vi "Get Modbus Channels.vi"(8 "error in (no error)":errorcluster, 10 "Chassis Name":tag, 11 "TimingGrp.lvclass":refnum<class "TimingGrp.lvclass">) -> (0 "error out":errorcluster, 1 "Num of Chans":i32, 3 "All Rate MB Chans":string[](array[string]))   [LabVIEW 2018, in "Configuration Grandmaster.lvlib" / "TimingGrp.lvclass"]
uses:
  TimingGrp.lvclass
  TimingGrp.lvclass/TimingGrp.ctl
  Class Chan Group/Read GroupChans.vi
  Measurements/Class Channel/Read ChanName.vi
  Measurements/Class Channel/Read ToModBus.vi
  Measurements/Class Channel/Channel.lvclass
  Class Chan Group/ChanGrp.lvclass
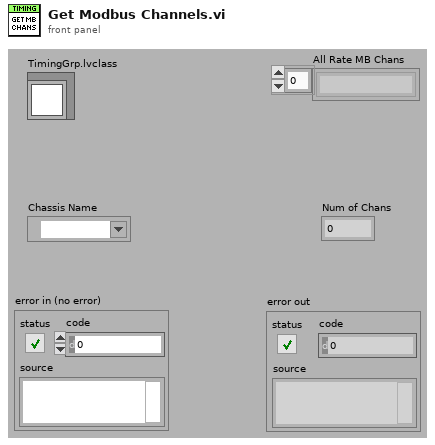
[diagram p1: front panel]
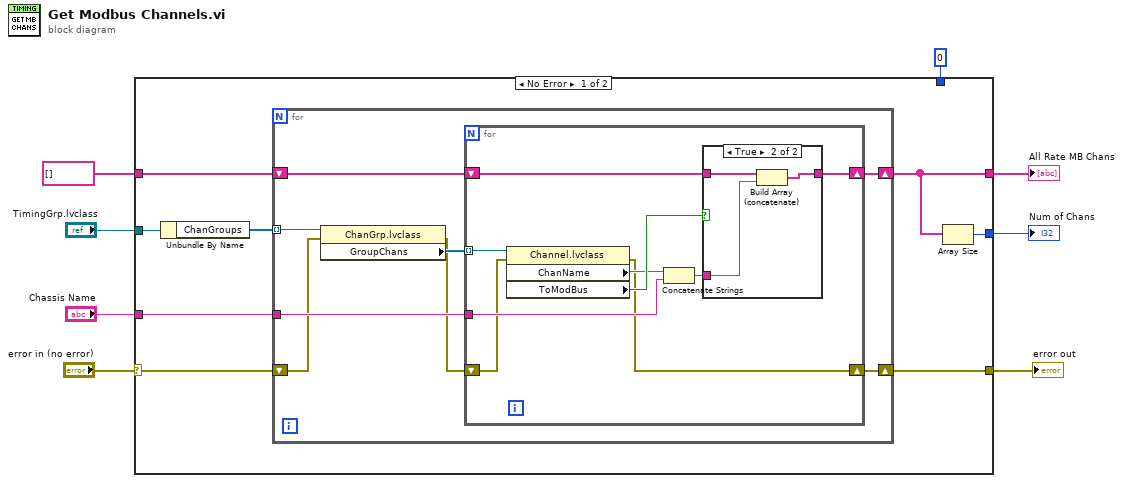
[diagram p0: block diagram]
diagram:
  n1 = case shown="No Error" "error in (no error)" {
    selector: "error in (no error)" -> [w9 w39]
    tunnel: string[] [] ("Grp Chans") -> [w16 w40]
    tunnel: [w15 w38] -> w7
    tunnel: [w14 w40] -> w6
    tunnel: "Chassis Name" -> [w13 _]
    tunnel: "TimingGrp.lvclass" -> [w12 _]
    tunnel: [w10 w39] -> w3
    tunnel: 0 -> [_ w38]
    frame No Error {
      n2 = Unbundle By Name(w12) -> ("ChanGroups"=w11:refnum<class "ChanGrp.lvclass">[])
      n3 = for {
        shift-right: [w23] -> w14
        shift-left: w16 -> [w24]
        tunnel: w13 -> [w20]
        tunnel: w11 -> [w22] mode=indexing
        shift-right: [w17] -> w10
        shift-left: w9 -> [w19]
        n4 = property class="ChanGrp.lvclass"(reference=w22, error in=w19) -> (error out=w18:errorcluster, "GroupChans"=w21:refnum<class "Channel.lvclass">[])  [unwired: 1 out]
        n5 = for {
          tunnel: w21 -> [w31] mode=indexing
          shift-right: [w32] -> w23
          shift-left: w24 -> [w33]
          tunnel: w20 -> [w27]
          shift-right: [w25] -> w17
          shift-left: w18 -> [w26]
          n6 = property class="Channel.lvclass"(reference=w31, error in=w26) -> (error out=w25:errorcluster, "ChanName"=w29:string, "ToModBus"=w30:bool)  [unwired: 1 out]
          n7 = Concatenate Strings(w29, w27) -> (w28:string)
          n8 = case shown="True" w30 {
            tunnel: w33 -> [w34 w37]
            tunnel: w28 -> [_ w36]
            tunnel: [w34 w35] -> w32
            frame False {
            }
            frame True {
              n9 = Build Array (concatenate)(w37, w36) -> (w35:string[])
            }
          }
        }
      }
      n10 = Array Size(array=w14) -> (size(s)=w15:i32)
    }
    frame Error {
    }
  }
  "All Rate MB Chans" <- w6
  "Num of Chans" <- w7
  "error out" <- w3
